vi "Append to Buffer.vi"(8 "error in":errorcluster, 9 "Level":dbl, 10 "Ident":string, 11 "BufferWrites1SamDBL in":refnum<class "BufferWrites1SamDBL.lvclass">) -> (0 "error out":errorcluster, 3 "BufferWrites1SamDBL out":refnum<class "BufferWrites1SamDBL.lvclass">)   [LabVIEW 2023, in "BufferWrites1SamDBL.lvclass"]
uses:
  BufferWrites1SamDBL.lvclass
  BufferWrites1SamDBL.lvclass/BufferWrites1SamDBL.ctl
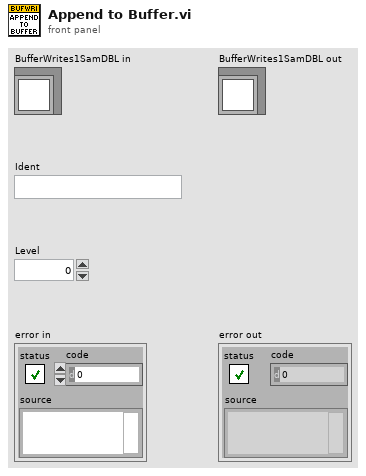
[diagram p1: front panel]
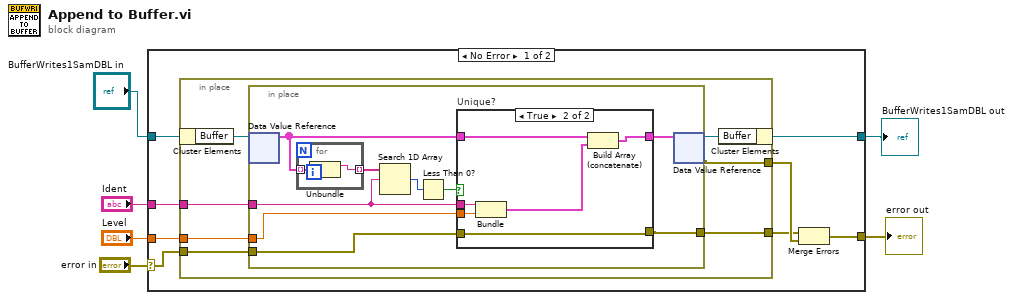
[diagram p0: block diagram]
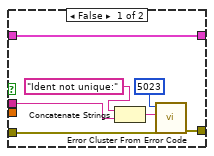
[diagram p2: hidden frame]
diagram:
  n1 = case shown="No Error" "error in" {
    selector: "error in" -> [w8 w47]
    tunnel: [w12 w47] -> w5
    tunnel: [w10 w46] -> w3
    tunnel: "BufferWrites1SamDBL in" -> [w14 w46]
    tunnel: "Level" -> [w13 _]
    tunnel: "Ident" -> [w9 _]
    frame No Error {
      n2 = in-place {
        in-place-border: w13 -> [w20]
        in-place-border: [w19] -> w11
        in-place-border: w9 -> [w17]
        in-place-border: w8 -> [w16]
        in-place-border: [w15] -> w7
        n3 = in-place-cluster #1(w14) -> ("Buffer"=w21:refnum<data-value>)
        n4 = in-place {
          in-place-border: w20 -> [w29]
          in-place-border: w17 -> [w22]
          in-place-border: w16 -> [w24]
          in-place-border: [w23] -> w15
          n5 = in-place-dvr #2(w21) -> (w28:cluster{"Ident":string, "Value":dbl}[])  [unwired: 1 out]
          n6 = for {
            tunnel: w28 -> [w44] mode=indexing
            tunnel: [w45] -> w27 mode=indexing
            n7 = Unbundle(w44) -> ("Ident"=w45:string)  [unwired: 1 out]
          }
          n8 = Search 1D Array(1D array=w27, element=w22) -> (index of element=w25:i32)  [unwired: 1 in]
          n9 = Less Than 0?(x=w25) -> (x < 0?=w26:bool)
          n10 = case "Unique?" shown="True" w26 {
            tunnel: w28 -> [w31 w43]
            tunnel: [w31 w42] -> w30
            tunnel: w22 -> [w32 w41]
            tunnel: w29 -> [_ w40]
            tunnel: w24 -> [w37 w38]
            tunnel: [w36 w38] -> w23
            frame False {
              n11 = Concatenate Strings("Ident not unique:" ("string"), w32) -> (w34:string)
              n12 = call <vilib>:"Error Cluster From Error Code.vi"("error in (no error)"=w37, "error message (\"\")"=w34, "error code (0)"=5023) -> ("error out"=w36:errorcluster)  [unwired: 6 in]
            }
            frame True {
              n13 = Bundle("Ident"=w41, "Level"=w40) -> (w39:cluster{"Ident":string, "Level":dbl})  [unwired: 1 in]
              n14 = Build Array (concatenate)(w43, w39) -> (w42:cluster{"Ident":string, "Level":dbl}[])
            }
          }
          n15 = in-place-dvr #2(w30) -> (w18:refnum<data-value>, w19:errorcluster)
        }
        n16 = in-place-cluster #1("Buffer"=w18) -> (w10:refnum<class "BufferWrites1SamDBL.lvclass">)
      }
      n17 = Merge Errors(w7, w11) -> (w12:errorcluster)
    }
    frame Error {
    }
  }
  "error out" <- w5
  "BufferWrites1SamDBL out" <- w3
